vi "Labview_diagram_nhom_10.vi"() -> ()   [LabVIEW 2020]
uses:
  <vilib>/Instr/_visa.llb/VISA Configure Serial Port (Instr).vi
panel:
  out "Alarm Light":bool
  out "NumBer People in the room":i32
  in  "VISA Port name":refnum<visa-resource-name>
  in  "?":bool
  out "Read buffer":string
  out "Lighting":bool
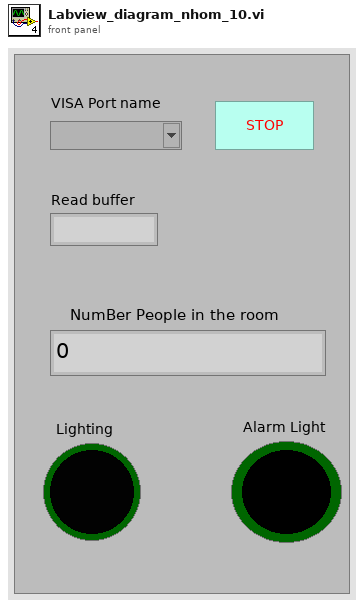
[diagram p1: front panel]
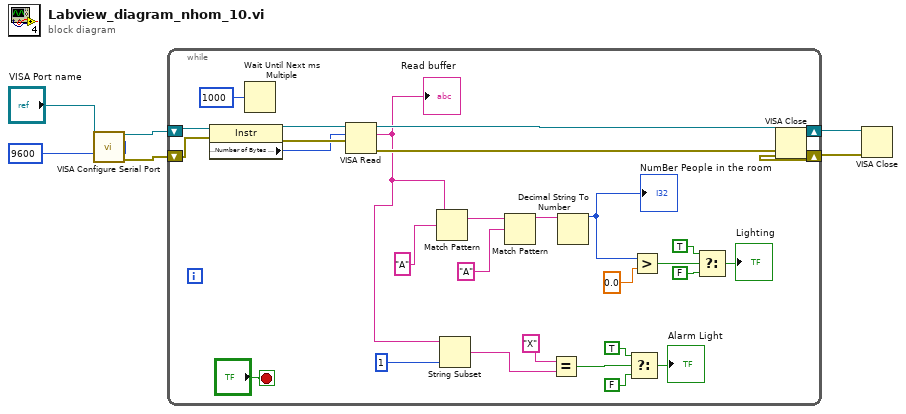
[diagram p0: block diagram]
diagram:
  n1 = call-poly "VISA Configure Serial Port"("VISA resource name"="VISA Port name", "baud rate (9600)"=u32 9600) -> ("VISA resource name out"=w6:refnum<visa-resource-name>, "error out"=w5:errorcluster)  [unwired: 12 in]
  n2 = while {
    shift-right: [w22] -> w2
    shift-left: w6 -> [w16]
    shift-right: [w28] -> w1
    shift-left: w5 -> [w17]
    stop <- "?" stop-if-true
    n3 = property class="Instr"(reference=w16, error in=w17) -> (reference out=w31:refnum<visa-resource-name>, error out=w32:errorcluster, "Serial Settings:Number of Bytes at Serial Port"=w30:u32)
    n4 = Wait Until Next ms Multiple(millisecond multiple=u32 1000) -> ()  [unwired: 1 out]
    n5 = VISA Read(VISA resource name=w31, byte count=w30, error in (no error)=w32) -> (VISA resource name out=w22:refnum<visa-resource-name>, read buffer=w9:string, error out=w28:errorcluster)  [unwired: 1 out]
    "Read buffer" <- w9
    n6 = Match Pattern(string=w9, regular expression="A") -> (after substring=w14:string)  [unwired: 1 in, 3 out]
    n7 = String Subset(string=w9, length (rest)=1 ("length (rest)")) -> (substring=w7:string)  [unwired: 1 in]
    n8 = Match Pattern(string=w14, regular expression="A") -> (before substring=w10:string)  [unwired: 1 in, 3 out]
    n9 = Equal?(x="X", y=w7) -> (x = y?=w18:bool)
    n10 = Decimal String To Number(string=w10) -> (number=w11:i32)  [unwired: 2 in, 1 out]
    "NumBer People in the room" <- w11
    n11 = Select(t=TRUE, s=w18, f=FALSE) -> (s? t:f=→"Alarm Light":bool)
    n12 = Greater?(x=w11, y=0.0) -> (0:w26:bool)
    n13 = Select(t=TRUE, s=w26, f=FALSE) -> (s? t:f=→"Lighting":bool)
  }
  n14 = VISA Close(VISA resource name=w2, error in (no error)=w1) -> ()  [unwired: 1 out]
  n15 = VISA Close(VISA resource name=w2, error in (no error)=w1) -> ()  [unwired: 1 out]
